vi "Run2 Toy factory.vi"(11 "NXT/EV3":T1) -> (3 "EV3 out":T1)   [LabVIEW 2016]
uses:
  <vilib>/NXT/Subs/LVHSConnector.ctl
  <vilib>/NXT/LegoClasses/BrickReference/BrickReference.lvclass
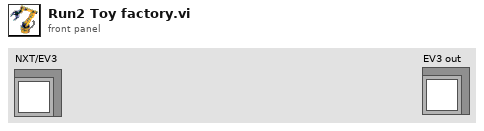
[diagram p1: front panel]
types:
  T1 = typedef "LVHSConnector.ctl" = refnum<class "BrickReference.lvclass">
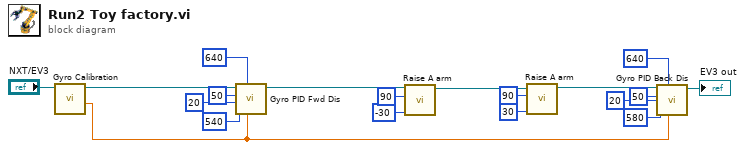
[diagram p0: block diagram]
diagram:
  n1 = call "Gyro Calibration.vi"("NXT/EV3"="NXT/EV3") -> ("Degrees"=w7:sgl, "NXT/EV3"=w19:T1)  [unwired: 6 in, 1 out]
  n2 = call "Gyro PID Fwd Dis.vi"("Target angle"=w7, "Threshold to stop"=640, "Threshold to slow"=540, "Min. speed"=20, "Max. speed"=50, "EV3 in"=w19) -> ("EV3 out"=w14:T1)  [unwired: 5 in]
  n3 = call "Raise A arm.vi"("Power"=i8 -30, "Rotation"=90, "EV3 in"=w14) -> ("EV3 out"=w4:T1)  [unwired: 8 in]
  n4 = call "Raise A arm.vi"("Power"=i8 30, "Rotation"=90, "EV3 in"=w4) -> ("EV3 out"=w3:T1)  [unwired: 8 in]
  n5 = call "Gyro PID Back Dis.vi"("Target angle"=w7, "Threshold to stop"=640, "Threshold to slow"=580, "Min. speed"=20, "Max. speed"=50, "EV3 in"=w3) -> ("EV3 out"=→"EV3 out":T1)  [unwired: 5 in]
